vi "Get Column Width.vi"(8 "error in":errorcluster, 10 "Column":i32, 11 "Sourcegrid in":refnum<class "SourceGrid.lvclass">) -> (0 "error out":errorcluster, 2 "Width":i32, 3 "Sourcegrid out":refnum<class "SourceGrid.lvclass">)   [LabVIEW 2023, in "SourceGrid.lvlib" / "SourceGrid.lvclass"]
uses:
  SourceGrid.lvclass
  SourceGrid.lvclass/SourceGrid.ctl
  D:/git/Sourcegrid-LabVIEW/dll/SourceGrid.dll
  dll/SourceGrid.dll
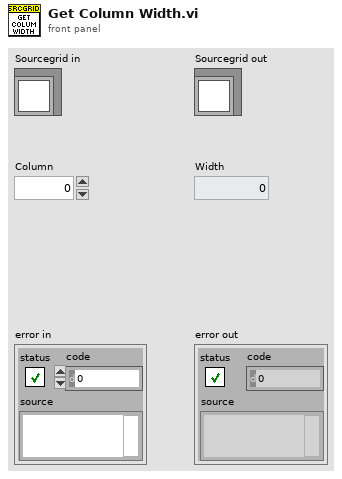
[diagram p1: front panel]
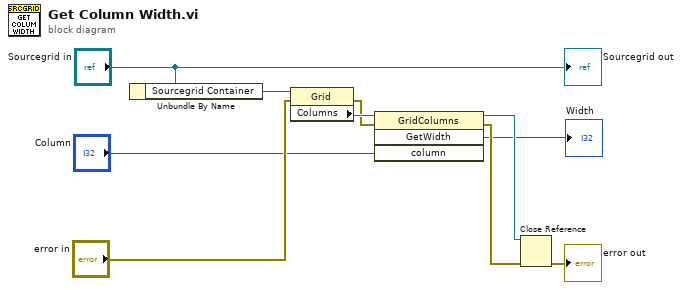
[diagram p0: block diagram]
diagram:
  n1 = Unbundle By Name("Sourcegrid in") -> ("Sourcegrid Container"=w7:refnum<k24>)
  n2 = property class="Grid"(reference=w7, error in="error in") -> (error out=w9:errorcluster, "Columns"=w10:refnum<k24>)  [unwired: 1 out]
  n3 = invoke class="GridColumns" method="GetWidth"(reference=w10, error in=w9, "column"="Column") -> (reference out=w3:refnum<k24>, error out=w5:errorcluster, "GetWidth"=→"Width":i32)  [unwired: 1 in, 1 out]
  n4 = Close Reference(reference=w3, error in (no error)=w5) -> (error out=→"error out":errorcluster)
  "Sourcegrid out" <- "Sourcegrid in"
